vi "Prep Command Info for Wait.vi"(6 "Synchronication":enum16{"Start", "Wait"}(ring), 8 "Command Info":T1) -> (0 "Command Info":T1, 1 "Allocated":bool)   [LabVIEW 2025]
doc: "If needed, create the Notifier that can ber used for synchronization. This is needed if this command is supposed to wait for completion and one wasn't created and passed in by upstream commands."
uses:
  <vilib>/Rock Robotics/WPI/Framework/Command Status Info.ctl
  <vilib>/Rock Robotics/WPI/Framework/Completion Status.ctl
  <vilib>/Rock Robotics/WPI/Framework/Completion Notifier.ctl
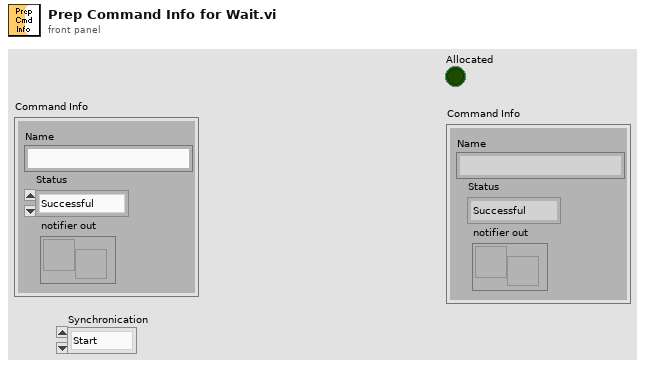
[diagram p1: front panel]
types:
  T1 = typedef "Command Status Info.ctl" = cluster{"Name":string, "Status":T2, "notifier out":T3}
  T2 = typedef "Completion Status.ctl" = enum16{"Successful", "Aborted", "Incomplete"}
  T3 = typedef "Completion Notifier.ctl" = refnum<notifier>
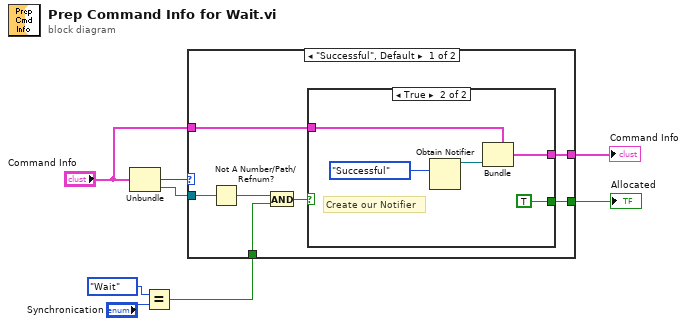
[diagram p0: block diagram]
diagram:
  n1 = Unbundle("Command Info") -> ("Status"=w5:T2, "notifier out"=w8:T3)  [unwired: 1 out]
  n2 = Equal?(x=enum16{"Start", "Wait"}."Wait" ("Synchronication"), y="Synchronication") -> (x = y?=w1:bool)
  n3 = case shown="\"Successful\", Default" w5 {
    tunnel: w8 -> [w15 _]
    tunnel: "Command Info" -> [w14 w22]
    tunnel: [w13 w22] -> w6
    tunnel: [w12 _] -> w4
    tunnel: w1 -> [w11 _]
    frame "Successful", Default {
      n4 = Not A Number/Path/Refnum?(number/path/refnum=w15) -> (NaN/Path/Refnum?=w10:bool)
      n5 = And(x=w10, y=w11) -> (x .and. y?=w9:bool)
      n6 = case shown="True" w9 {
        tunnel: w14 -> [w16 w20]
        tunnel: [w16 w18] -> w13
        tunnel: [_ TRUE] -> w12
        frame False {
          # "Reuse the existing command\nNotifier"
        }
        frame True {
          # "Create our Notifier"
          n7 = Obtain Notifier(notification data type=Completion_Status."Successful") -> (notifier out=w19:refnum<notifier>)  [unwired: 3 in, 2 out]
          n8 = Bundle(cluster=w20, "notifier out"=w19) -> (w18:T1)  [unwired: 2 in]
        }
      }
    }
    frame "Aborted" {
    }
  }
  "Command Info" <- w6
  "Allocated" <- w4
